vi "Destroy Events.vi"(8 "error in (no error)":errorcluster, 11 "SMO":refnum<class "SMO.lvclass">) -> (0 "error out":errorcluster, 3 "SMO out":refnum<class "SMO.lvclass">)   [LabVIEW 2013, in "SMO.lvclass"]
uses:
  SMO.lvclass
panel:
  # "For instructions on how to use the JKI State Machine Objects, examples and video tutorials, visit:\nhttp://jki.net/state-machine-objects/\n\nJKI State Machine Objects™\nhttp://jki.net/state-machine-objects/\nCopyright (C) 2005-2015, JKI <info@jki.net>\nALL RIGHTS RESERVED"
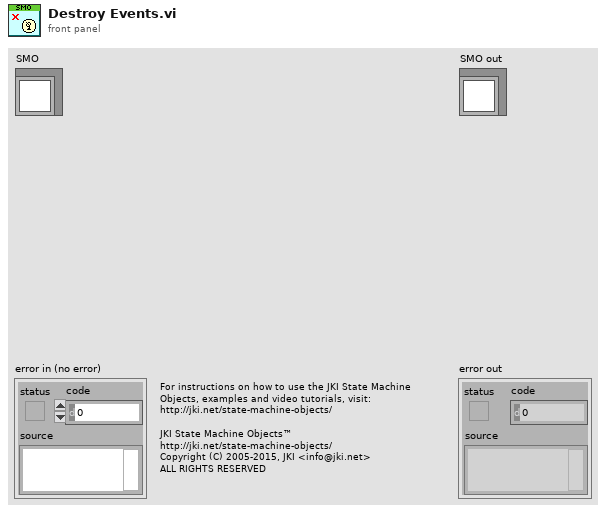
[diagram p1: front panel]
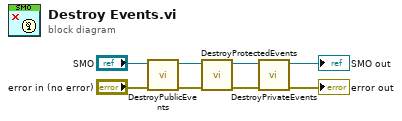
[diagram p0: block diagram]
diagram:
  n1 = call-dynamic "DestroyPublicEvents.vi"("error in (no error)"="error in (no error)", "SMO"="SMO") -> ("error out"=w6:errorcluster, "SMO out"=w5:refnum<class "SMO.lvclass">)  [unwired: 8 in]
  n2 = call-dynamic "DestroyProtectedEvents.vi"("error in (no error)"=w6, "SMO"=w5) -> ("error out"=w2:errorcluster, "SMO out"=w4:refnum<class "SMO.lvclass">)  [unwired: 8 in]
  n3 = call-dynamic "DestroyPrivateEvents.vi"("error in (no error)"=w2, "SMO"=w4) -> ("error out"=→"error out":errorcluster, "SMO out"=→"SMO out":refnum<class "SMO.lvclass">)  [unwired: 8 in]
